vi "settle_timer.vi"(0 "Temp":dbl, 7 "Control Parameters":T1={"Setpoint"=50.0, "Control bandwidth"=4.0, "Settle bandwidth"=1.0, "Integral time"=30.0, "Int\non"=TRUE, "Derivative time"=0.5, "Der\non"=TRUE, "Settle time"=60.0} {"Settle time" format="%.2f"; "Derivative time" format="%.2f"; "Integral time" format="%.2f"; "Settle bandwidth" format="%.2f"; "Control bandwidth" format="%.2f"; "Setpoint" format="%.2f"}, 13 "Elapsed Time":dbl) -> (4 "Settle Time":dbl, 8 "Settled":bool)   [LabVIEW 2016]
uses:
  typedefs/control parameters.ctl
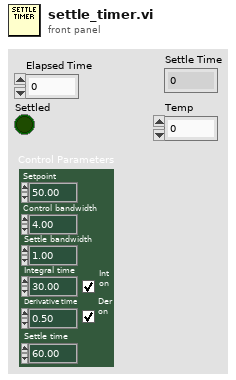
[diagram p1: front panel]
types:
  T1 = typedef "control parameters.ctl" = cluster{"Setpoint":dbl, "Control bandwidth":dbl, "Settle bandwidth":dbl, "Integral time":dbl, "Int\non":bool, "Derivative time":dbl, "Der\non":bool, "Settle time":dbl}
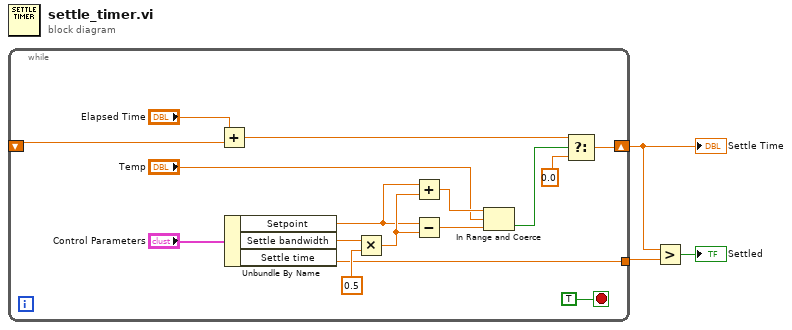
[diagram p0: block diagram]
diagram:
  n1 = while {
    tunnel: [w5] -> w2
    shift-right: [w9] -> w3
    shift-left: _ -> [w4]
    stop <- TRUE stop-if-true
    n2 = Add(x="Elapsed Time", y=w4) -> (x+y=w7:dbl)
    n3 = Unbundle By Name("Control Parameters") -> ("Setpoint"=w16:dbl, "Settle bandwidth"=w15:dbl, "Settle time"=w5:dbl)
    n4 = Multiply(x=w15, y=0.5) -> (x*y=w17:dbl)
    n5 = Add(x=w16, y=w17) -> (x+y=w14:dbl)
    n6 = Subtract(x=w16, y=w17) -> (x-y=w13:dbl)
    n7 = In Range and Coerce(upper limit=w14, x="Temp", lower limit=w13) -> (In Range?=w11:bool)  [unwired: 1 out]
    n8 = Select(t=w7, s=w11, f=0.0) -> (s? t:f=w9:dbl)
  }
  "Settle Time" <- w3
  n9 = Greater?(x=w3, y=w2) -> (0:→"Settled":bool)
